vi "InitClassTree.vi"(8 "error in (no error)":errorcluster, 10 "TreeStrict":refnum<vi>, 11 "ClassDataTree in":refnum<class "ClassDataTree.lvclass">) -> (0 "error out":errorcluster, 3 "ClassDataTree out":refnum<class "ClassDataTree.lvclass">)   [LabVIEW 2010, in "ClassDataTree.lvclass"]
uses:
  ClassDataTree.lvclass
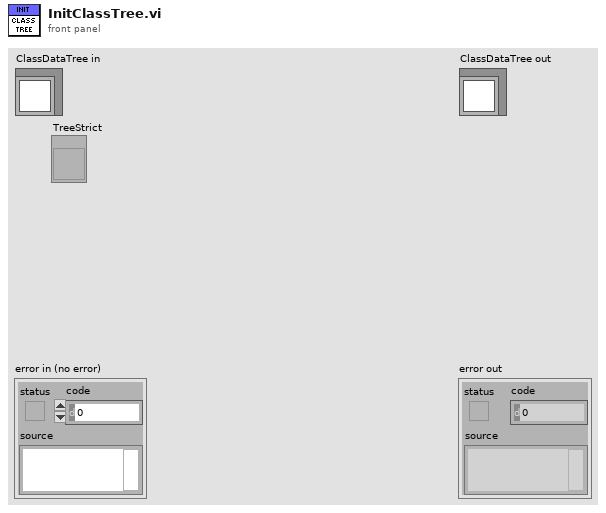
[diagram p1: front panel]
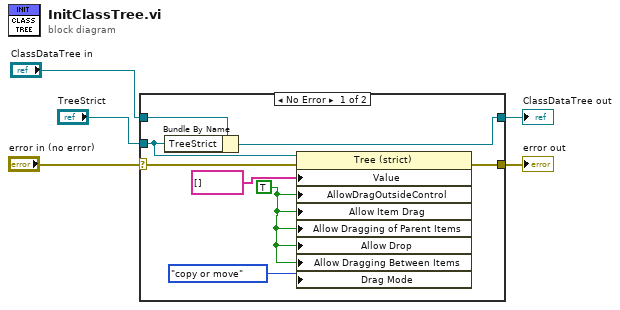
[diagram p0: block diagram]
diagram:
  n1 = case shown="No Error" "error in (no error)" {
    selector: "error in (no error)" -> [w13 w15]
    tunnel: [w12 w15] -> w4
    tunnel: "ClassDataTree in" -> [w11 w14]
    tunnel: [w10 w14] -> w2
    tunnel: "TreeStrict" -> [w9 _]
    frame No Error {
      w7 = TRUE ("Drag/Drop:Allow Dropping")
      n2 = Bundle By Name(cluster=w11, "TreeStrict"=w9) -> (w10:refnum<class "ClassDataTree.lvclass">)
      n3 = property class="Tree (strict)"(reference=w9, error in=w13, "Value"=string[] [], "AllowDragOutsideControl"=w7, "Allow Item Drag"=w7, "Allow Dragging of Parent Items"=w7, "Allow Drop"=w7, "Allow Dragging Between Items"=w7, "Drag Mode"=enum32{"copy or move", "copy only", "move only"}."copy or move" ("Drag/Drop:Drag Mode")) -> (error out=w12:errorcluster)  [unwired: 1 out]
    }
    frame Error {
    }
  }
  "error out" <- w4
  "ClassDataTree out" <- w2
